vi "LWXPS_GatheringRun.vi"(6 "LabVIEW error IN":errorcluster, 7 "Divisor":i32, 8 "Data Number":i32, 9 "XPS Reference IN":refnum<k24>) -> (0 "LabVIEW error OUT":errorcluster, 1 "XPS Error String":string, 2 "Returned error code":i32, 3 "XPS Reference OUT":refnum<k24>)   [LabVIEW 2014]
uses:
  D:/XPSQ8_LabView_Library/Development/Source/Dll/Newport.XPS.CommandInterface.dll
  Dll/Newport.XPS.CommandInterface.dll
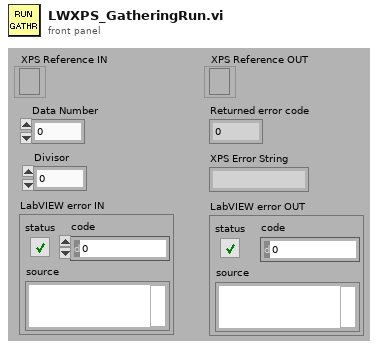
[diagram p1: front panel]
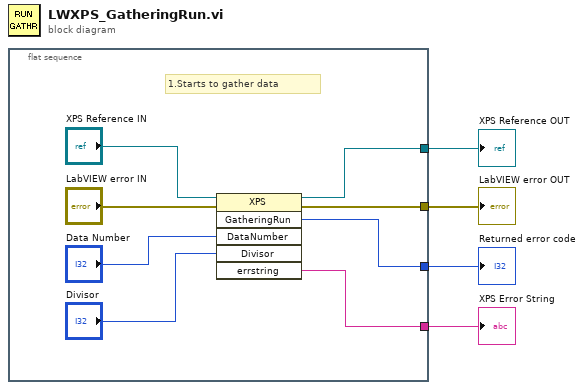
[diagram p0: block diagram]
diagram:
  n1 = flat-sequence {
    tunnel: [w11] -> w4
    tunnel: [w10] -> w3
    tunnel: [w9] -> w2
    tunnel: [w7] -> w1
    frame #0 {
      # "1.Starts to gather data"
      n2 = invoke class="XPS" method="GatheringRun"(reference="XPS Reference IN", error in="LabVIEW error IN", "DataNumber"="Data Number", "Divisor"="Divisor") -> (reference out=w11:refnum<k24>, error out=w10:errorcluster, "GatheringRun"=w9:i32, "errstring"=w7:string)  [unwired: 2 in, 2 out]
    }
  }
  "XPS Reference OUT" <- w4
  "LabVIEW error OUT" <- w3
  "Returned error code" <- w2
  "XPS Error String" <- w1
